vi "AzCamParse.vi"(0 "InputString":string="OK arg1 arg2 arg3 arg4") -> (1 "Error":bool, 2 "Reply":string="arg4")   [LabVIEW 2014]
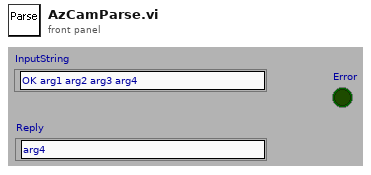
[diagram p1: front panel]
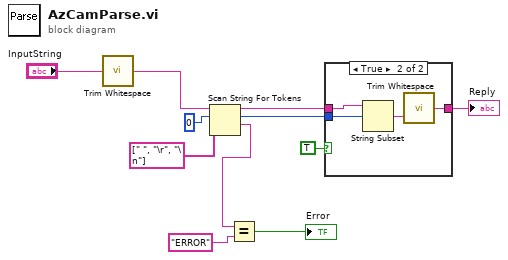
[diagram p0: block diagram]
diagram:
  n1 = call <vilib>:"Trim Whitespace.vi"("string"="InputString") -> ("trimmed string"=w1:string)  [unwired: 1 in]
  n2 = Scan String For Tokens(6:string[] [" ", "\r", "\n"] ("delimiters (\\s,\\t,\\r,\\n)"), 8:0 ("offset"), 9:w1) -> (1:w5:string, 2:w8:i32, 3:w7:string)  [unwired: 3 in, 1 out]
  n3 = Equal?(x=w5, y="ERROR") -> (x = y?=→"Error":bool)
  n4 = case shown="True" TRUE {
    tunnel: w8 -> [_ w16]
    tunnel: w7 -> [w12 w15]
    tunnel: [w12 w13] -> w6
    frame False {
    }
    frame True {
      n5 = String Subset(string=w15, offset (0)=w16) -> (substring=w14:string)  [unwired: 1 in]
      n6 = call <vilib>:"Trim Whitespace.vi"("string"=w14) -> ("trimmed string"=w13:string)  [unwired: 1 in]
    }
  }
  "Reply" <- w6
